vi "NIIE_Remove invalid characters.vi"(11 "String in":string) -> (3 "Filtered string out":string)   [LabVIEW 2021]
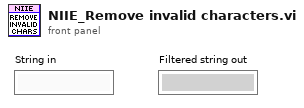
[diagram p1: front panel]
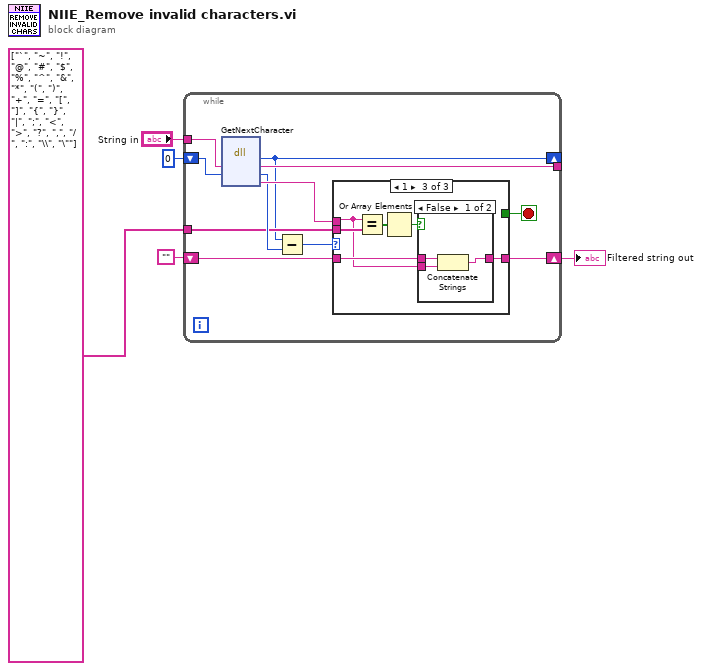
[diagram p0: block diagram]
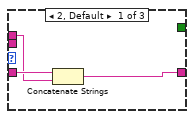
[diagram p2: hidden frame]
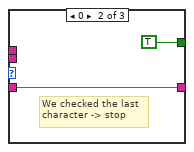
[diagram p3: hidden frame]
diagram:
  n1 = while {
    tunnel: [w16] -> _
    shift-right: [w6] -> _
    shift-left: 0 ("return type") -> [w15]
    shift-right: [w11] -> w1
    shift-left: "" -> [w13]
    tunnel: "String in" -> [w14]
    tunnel: string[] ["`", "~", "!", "@", "#", "$", "%", "^", "&", "*", "(", ")", "+", "=", "[", "]", "{", "}", "|", ";", "<", ">", "?", ",", "/", ":", "\\", "\""] -> [w8]
    stop <- w7 stop-if-true
    n2 = dll-call lib="LabVIEW" fn="GetNextCharacter"("string"=w14, "offset"=w15) -> ("return type"=w6:i32, "string"=w16:string, "offset"=w10:i32, "nextChar"=w12:string)  [unwired: 3 in, 3 out]
    n3 = Subtract(x=w6, y=w10) -> (x-y=w9:i32)
    n4 = case shown="1" w9 {
      tunnel: w13 -> [w19 w21 w24]
      tunnel: w12 -> [w18 _ w22]
      tunnel: [w17 w21 w23] -> w11
      tunnel: w8 -> [_ _ w27]
      tunnel: [_ TRUE _] -> w7
      frame 2, Default {
        n5 = Concatenate Strings(w19, w18) -> (w17:string)
      }
      frame 0 {
        # "We checked the last\ncharacter -> stop"
      }
      frame 1 {
        n6 = Equal?(x=w22, y=w27) -> (x = y?=w26:bool[])
        n7 = Or Array Elements(Boolean array=w26) -> (logical OR=w25:bool)
        n8 = case shown="False" w25 {
          tunnel: w24 -> [w30 w31]
          tunnel: [w29 w31] -> w23
          tunnel: w22 -> [w28 _]
          frame False {
            n9 = Concatenate Strings(w30, w28) -> (w29:string)
          }
          frame True {
          }
        }
      }
    }
  }
  "Filtered string out" <- w1
